vi "XIPIN_10G_Ethernet_PCS_PMA_(10GBASE-R_KR)_6_0.vi"   [LabVIEW 2017]
doc: "The Xilinx 10 Gigabit Ethernet PCS/PMA (10GBASE-R/KR) core is designed to the IEEE specification 802.3 2012. An example design is provided to accelerate your design cycle.\n------------------------------------\n<b>Need License</b> : Yes"
uses:
  <vilib>/rvi/XilinxIP/XIPIN_XNode/niFpgaXIPIN.xnode
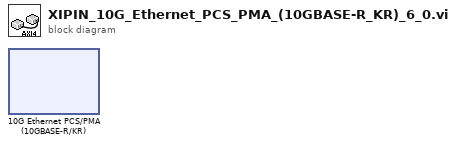
[diagram p0: block diagram]
diagram:
  n1 = xnode ("10G Ethernet PCS/PMA (10GBASE-R/KR)")() -> ()
